vi "Write FPENs.vi"(3 "FP":refnum<class "DecFrame_FP.lvclass">, 4 "FPEN":refnum<class "FPEN.lvclass">) -> (5 "FP Out":refnum<class "DecFrame_FP.lvclass">)   [LabVIEW 2023, in "DecFrame_FP.lvclass"]
uses:
  DecFrame_FP/DecFrame_FP.lvclass
  FPEN/FPEN.lvclass
  DecFrame_FP/DecFrame_FP.lvclass/DecFrame_FP.ctl
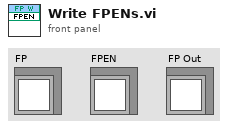
[diagram p1: front panel]
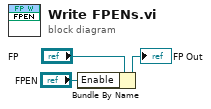
[diagram p0: block diagram]
diagram:
  n1 = Bundle By Name(cluster="FP", "Enable"="FPEN") -> (→"FP Out":refnum<class "DecFrame_FP.lvclass">)
